vi "Log.vi"(7 "Source":string, 8 "error in (no error)":errorcluster, 9 "Message":string, 10 "Level":T1, 11 "Mock Log Handler In":refnum<class "Mock Log Handler.lvclass">) -> (0 "error out":errorcluster, 3 "Mock Log Handler Out":refnum<class "Mock Log Handler.lvclass">)   [LabVIEW 2020, in "Mock Log Handler.lvclass"]
doc: "Enter a message into the system log."
uses:
  Mock Log Handler.lvclass
  Framework/Logging/Protected/Level.ctl
  Private/Log Entry.ctl
  Mock Log Handler.lvclass/Mock Log Handler.ctl
  Framework/Logging/Logging.lvclass
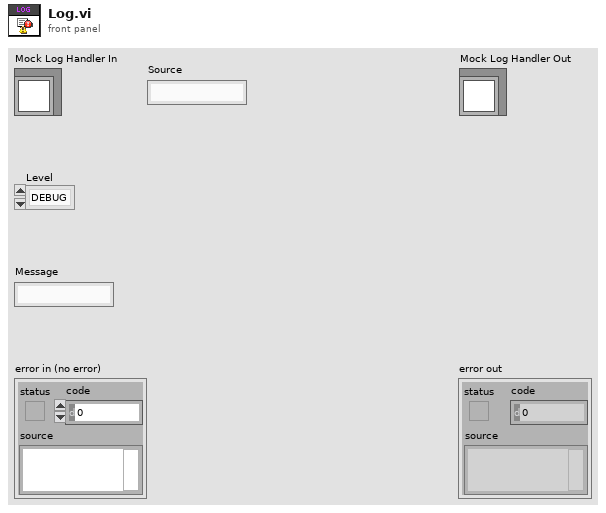
[diagram p1: front panel]
types:
  T1 = typedef "Logging.lvclass/Level.ctl" = enum16{"DEBUG", "INFO", "WARNING", "ERROR", "CRITICAL"}
  T2 = typedef "Mock Log Handler.lvclass/Log Entry.ctl" = cluster{"Level":string, "Source":string, "Message":string}
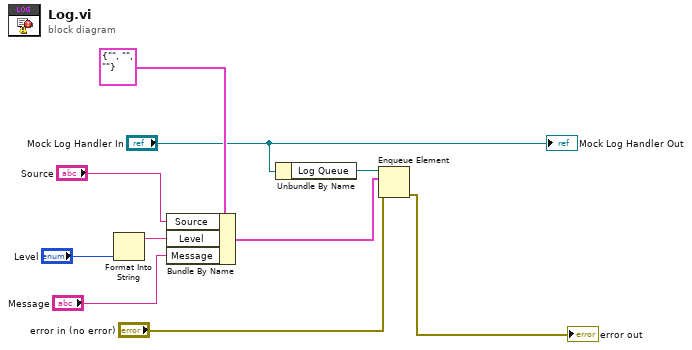
[diagram p0: block diagram]
diagram:
  n1 = Format Into String("Level") -> (resulting string=w6:string)  [unwired: 3 in, 1 out]
  n2 = Bundle By Name(cluster=T2 {"Level"="", "Source"="", "Message"=""} ("Cluster"), "Source"="Source", "Level"=w6, "Message"="Message") -> (w3:T2)
  n3 = Unbundle By Name("Mock Log Handler In") -> ("Log Queue"=w4:refnum<queue>)
  n4 = Enqueue Element(queue=w4, element=w3, error in (no error)="error in (no error)") -> (error out=→"error out":errorcluster)  [unwired: 1 in, 2 out]
  "Mock Log Handler Out" <- "Mock Log Handler In"
